vi "Running Histogram.vi"() -> ()   [LabVIEW 2023]
doc: "Uses the General Histogram VI to implement a running histogram. This example generates continuous Gaussian noise, computes the histogram of the noise, and adds the new histogram to the sum of all the previous histograms. In addition to computing the histogram, the General Histogram VI also computes the number of points that are outside all bins. This example keeps a running total of this quantity. The bins of the histogram span three standard deviations of the noise level. The histogram plot should begin to resemble a Gaussian curve as more points are added to the histogram. The units of the histogram display are % of total points. \n\nNote: There is a Point by Point function palette which provides an easier way to implement a running histogram. See the Moving Histogram PtByPt.vi example for more information."
uses:
  <vilib>/Analysis/NI_AALPro.lvlib
  <vilib>/Analysis/NI_AALBase.lvlib
panel:
  out "# outside":cluster{"total":i32, "below":i32, "above":i32}
  in  "Averaging type":u16(ring)=1 items=["Linear", "Exponential"]
  in  "Exponential factor":dbl(slide)=0.9 min=0.01 max=0.999 step=0.01 scale=0.0..1.0
  in  "Mean value":dbl(slide) scale=-1.0..1.0
  in  "Noise level":dbl(knob)=0.5 scale=0.1..1.0
  out "Measurements":dbl[](graph)
  in  "Number of bins":i32=50
  in  "Stop":bool
  out "Histogram":cluster{"Histogram":dbl[], "Axis":dbl[]}[](graph)
  # "Overview: This VI demonstrates how to implement a running histogram using the General Histogram VI.\nRequirements: LabVIEW Full Development System\nInstructions:\n1. Run the VI.\n2. Set the Exponential Factor to a small value (close to 0), so the past histogram results contribute less to the running total. The Histogram will respond closely as you change the Mean value of noise parameters.\n3. Set the Exponential Factor to a larger value (close to 1), so the past histogram results contribute more to the running total. The Histogram will respond slowly to noise control changes.\n4. Click Stop to stop the VI."
  # "Noise Parameters"
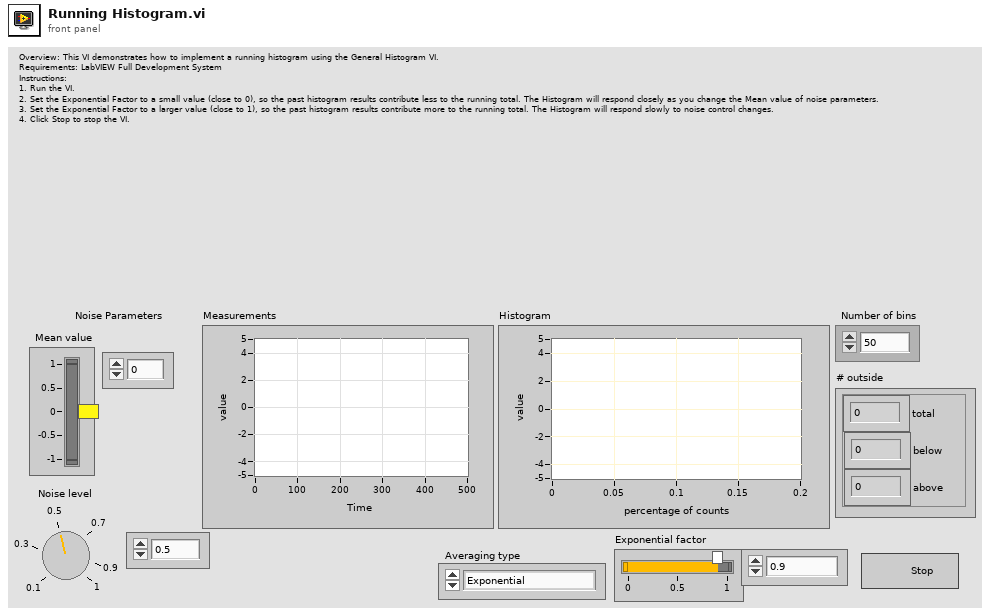
[diagram p1: front panel]
types:
  T1 = enum8{"Enabled", "Disabled", "Disabled and Grayed Out"}
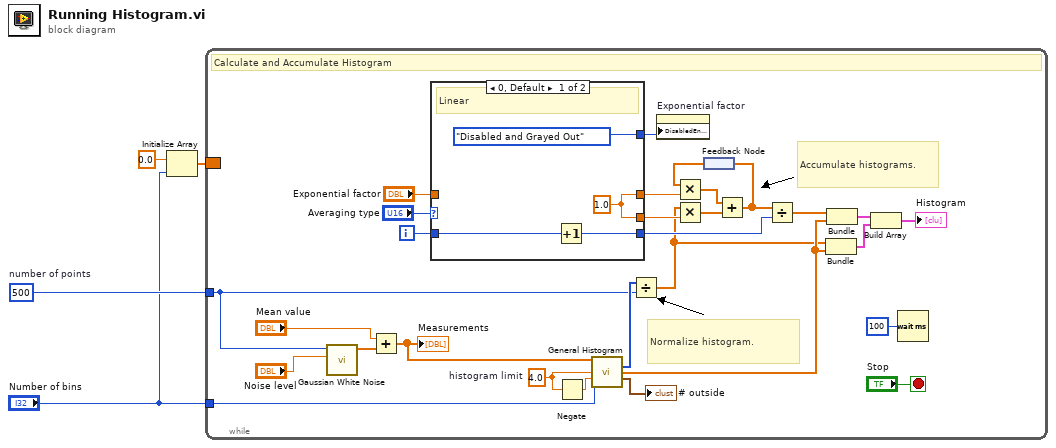
[diagram p0: block diagram]
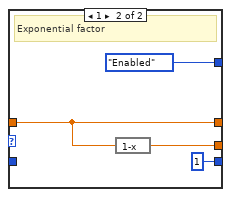
[diagram p2: hidden frame]
diagram:
  w4 = 500  # number of points
  n1 = Initialize Array(0.0, "Number of bins") -> (w1:dbl[])
  n2 = while {
    tunnel: "Number of bins" -> [w31]
    tunnel: w4 -> [w11]
    border: w1 -> [_]
    i -> [w6]
    stop <- "Stop" stop-if-true
    w20 = 4.0  # histogram limit
    # "Accumulate histograms."
    # "Normalize histogram."
    # "Calculate and Accumulate Histogram"
    n3 = call <vilib>:"Gaussian White Noise.vi"("standard deviation"="Noise level", "samples"=w11) -> ("Gaussian noise pattern"=w33:dbl[])  [unwired: 8 in, 1 out]
    n4 = Add(x="Mean value", y=w33) -> (x+y=w19:dbl[])
    "Measurements" <- w19
    n5 = case shown="0, Default" "Averaging type" {
      tunnel: [w37 w40] -> w15
      tunnel: "Exponential factor" -> [_ w40]
      tunnel: [w37 w39] -> w12
      tunnel: [w35 1 ("number of points")] -> w8
      tunnel: w6 -> [w36 _]
      tunnel: [T1."Disabled and Grayed Out" ("Disabled") T1."Enabled" ("Disabled")] -> w5
      frame 0, Default {
        w37 = 1.0
        # "Linear"
        n6 = Increment(x=w36) -> (x+1=w35:i32)
      }
      frame 1 {
        # "Exponential factor"
        n7 = expression code="1-x"(w40) -> (w39:dbl)
      }
    }
    n8 = Negate(x=w20) -> (-x=w27:dbl)
    n9 = call <vilib>:"General Histogram.vi"("X"=w19, "max"=w20, "min"=w27, "# bins"=w31) -> ("Histogram"=w24:i32[], "Axis"=w25:dbl[], "# outside"=→"# outside":cluster{"total":i32, "below":i32, "above":i32})  [unwired: 7 in, 2 out]
    n10 = Divide(x=w24, y=w11) -> (x/y=w7:dbl[])
    n11 = property on="Exponential factor" class="Slide (strict)"("DisabledEnum"=w5) -> ()  [unwired: 2 in, 2 out]
    n12 = Multiply(x=w7, y=w12) -> (x*y=w16:dbl[])
    n13 = feedback #1() -> (w32:dbl[])
    n14 = Multiply(x=w32, y=w15) -> (x*y=w17:dbl[])
    n15 = Add(x=w17, y=w16) -> (x+y=w10:dbl[])
    n16 = feedback-in #1(w10) -> ()
    n17 = Divide(x=w10, y=w8) -> (x/y=w9:dbl[])
    n18 = Bundle(w7, "Axis"=w25) -> (w22:cluster{dbl[], "Axis":dbl[]})  [unwired: 1 in]
    n19 = Bundle(w9, "Axis"=w25) -> (w23:cluster{dbl[], "Axis":dbl[]})  [unwired: 1 in]
    n20 = Build Array(w23, w22) -> (→"Histogram":cluster{dbl[], "Axis":dbl[]}[])
    n21 = Wait (ms)(milliseconds to wait=u32 100) -> ()  [unwired: 1 out]
  }
